vi "GetTotalSeqs.vi"(8 "error in (no error)":errorcluster, 11 "Channel in":refnum<class "Channel.lvclass">) -> (0 "error out":errorcluster, 3 "Channel out":refnum<class "Channel.lvclass">)   [LabVIEW 2018, in "Channel.lvclass"]
uses:
  Channel.lvclass
  Channel.lvclass/Channel.ctl
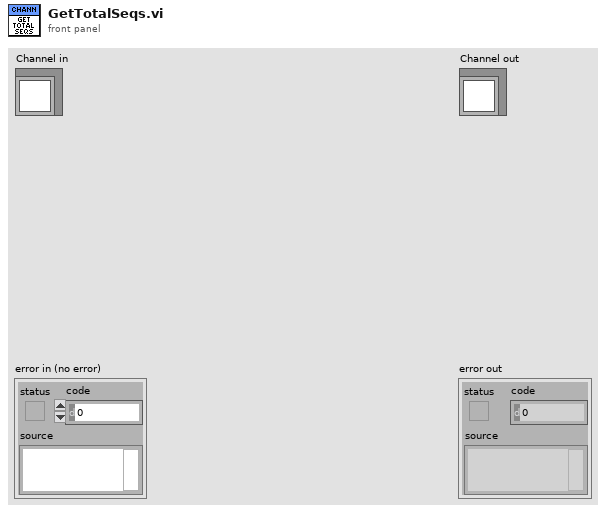
[diagram p1: front panel]
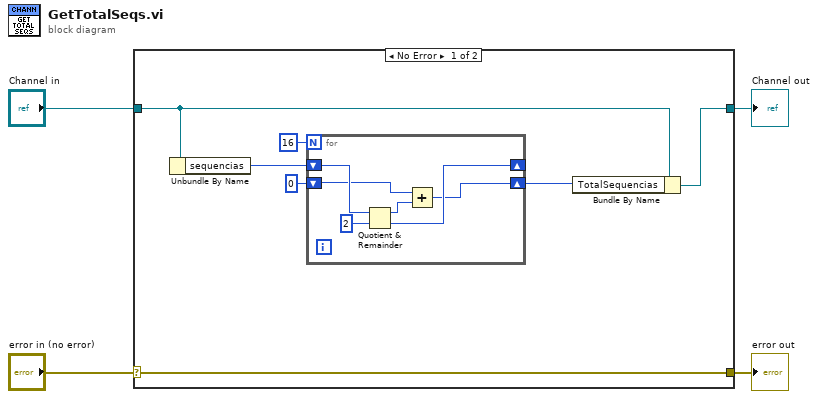
[diagram p0: block diagram]
diagram:
  n1 = case shown="No Error" "error in (no error)" {
    selector: "error in (no error)" -> [w11 w19]
    tunnel: [w11 w19] -> w3
    tunnel: [w7 w18] -> w1
    tunnel: "Channel in" -> [w8 w18]
    frame No Error {
      n2 = Unbundle By Name(w8) -> ("sequencias"=w9:u32)
      n3 = for {
        N: 16 -> [_]
        shift-right: [w15] -> _
        shift-left: w9 -> [w17]
        shift-right: [w12] -> w6
        shift-left: u32 0 -> [w13]
        n4 = Quotient & Remainder(x=w17, y=u32 2) -> (x-y*floor(x/y)=w14:u32, floor(x/y)=w15:u32)
        n5 = Add(x=w13, y=w14) -> (x+y=w12:u32)
      }
      n6 = Bundle By Name(cluster=w8, "TotalSequencias"=w6) -> (w7:refnum<class "Channel.lvclass">)
    }
    frame Error {
    }
  }
  "error out" <- w3
  "Channel out" <- w1
